vi "Wash Display.vi"(11 "Message Queues":T1) -> ()   [LabVIEW 2017]
uses:
  support/Message Queue/All Message Queues.ctl
  support/Message Queue/Message Cluster.ctl
  Control 1.ctl
  Position Slider.ctl
  support/Message Queue/Message Queue.lvlib
panel:
  out "Wash Entry Display":bool
  out "Vehicle Postion":bool
  out "Air Dry":bool
  out "Tire Shine Foam":bool
  out "Spot Free Rinse":bool
  out "Low Pressure  Wax":bool
  out "High Pressure Wash":bool
  out "Pre-soak":bool
  out "Bug Remover":bool
  out "Under Body Wash":bool
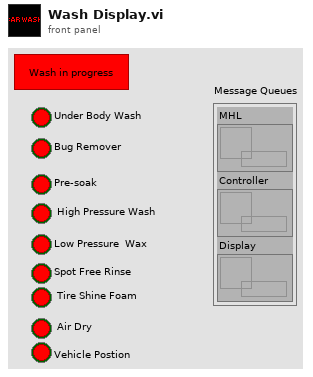
[diagram p1: front panel]
types:
  T1 = typedef "Message Queue.lvlib/All Message Queues.ctl" = cluster{"MHL":refnum<queue>, "Controller":refnum<queue>, "Display":refnum<queue>}
  T2 = typedef "Control 1.ctl" = cluster{"Under Body Wash":bool, "Bug Remover":bool, "Pre-soak":bool, " High Pressure Wash":bool, "Low Pressure  Wax":bool, "Spot Free Rinse":bool, " Tire Shine Foam":bool, " Air Dry":bool, "Vehicle Postion":bool, "Wash Entry Display":bool, "Car Position Slider":T3}
  T3 = typedef "Position Slider.ctl" = i32
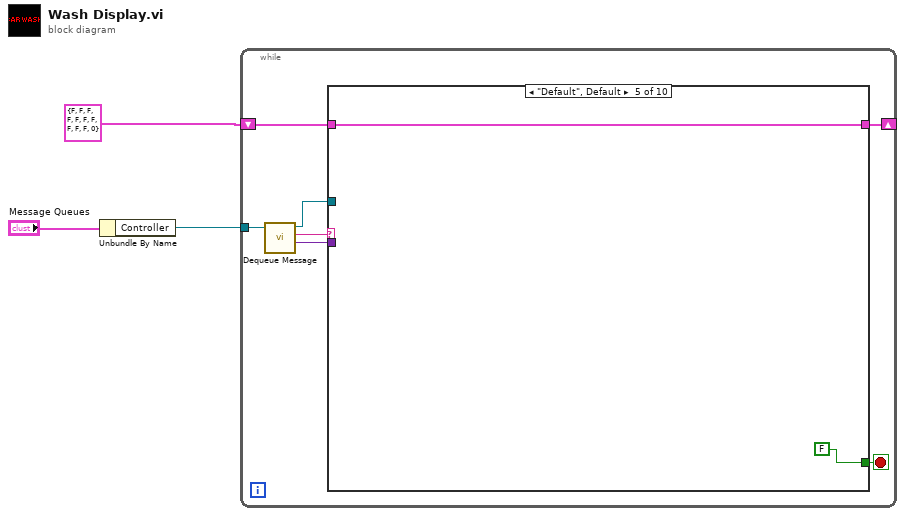
[diagram p0: block diagram]
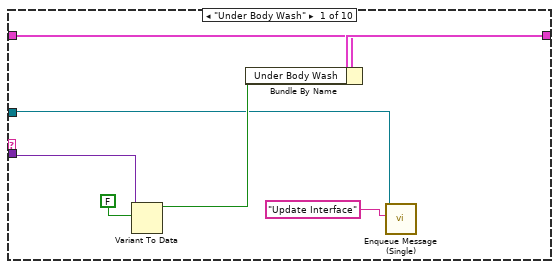
[diagram p2: hidden frame]
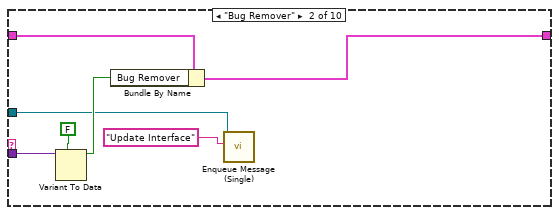
[diagram p3: hidden frame]
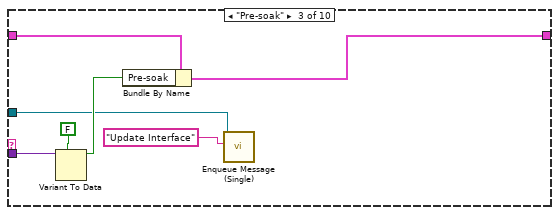
[diagram p4: hidden frame]
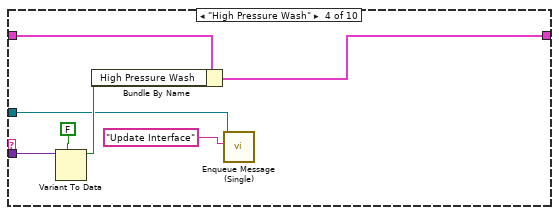
[diagram p5: hidden frame]
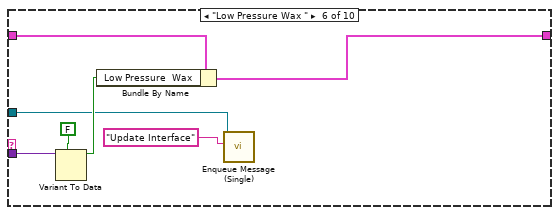
[diagram p6: hidden frame]
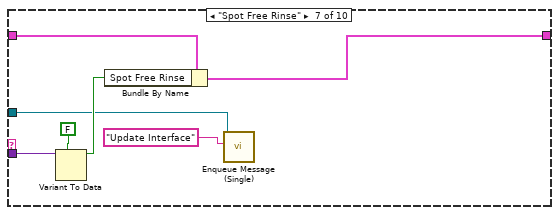
[diagram p7: hidden frame]
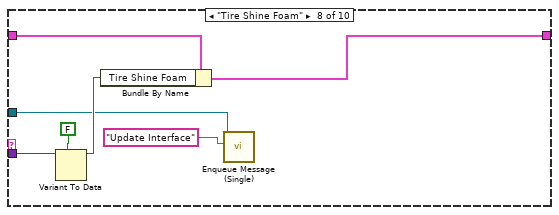
[diagram p8: hidden frame]
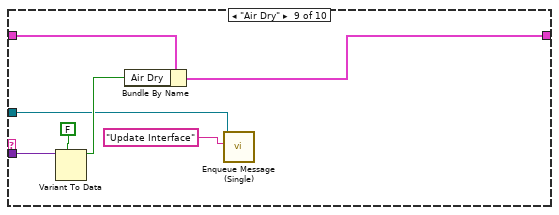
[diagram p9: hidden frame]
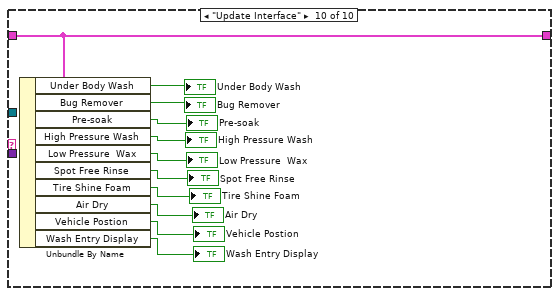
[diagram p10: hidden frame]
diagram:
  n1 = Unbundle By Name("Message Queues") -> ("Controller"=w2:refnum<queue>)
  n2 = while {
    tunnel: w2 -> [w10]
    shift-right: [w7] -> _
    shift-left: T2 {"Under Body Wash"=FALSE, "Bug Remover"=FALSE, "Pre-soak"=FALSE, " High Pressure Wash"=FALSE, "Low Pressure  Wax"=FALSE, "Spot Free Rinse"=FALSE, " Tire Shine Foam"=FALSE, " Air Dry"=FALSE, "Vehicle Postion"=FALSE, "Wash Entry Display"=FALSE, "Car Position Slider"=0} -> [w8]
    stop <- w4 stop-if-true
    n3 = call "Dequeue Message.vi"("Message Queue"=w10) -> ("Message Data"=w5:variant, "Message"=w9:string, "dup Message Queue"=w6:refnum<queue>)  [unwired: 7 in, 1 out]
    n4 = case shown="\"Default\", Default" w9 {
      tunnel: w8 -> [w11 w23 w30 w37 w40 w46 w53 w60 w67 w79]
      tunnel: [w14 w20 w27 w34 w40 w43 w50 w57 w64 w79] -> w7
      tunnel: w6 -> [w13 w19 w26 w33 _ w42 w49 w56 w63 _]
      tunnel: w5 -> [w17 w24 w31 w38 _ w47 w54 w61 w68 _]
      tunnel: [_ _ _ _ FALSE _ _ _ _ _] -> w4
      frame "Under Body Wash" {
        n5 = Variant To Data(type=FALSE, Variant=w17) -> (data=w16:bool)  [unwired: 1 in, 1 out]
        n6 = Bundle By Name(cluster=w11, "Under Body Wash"=w16) -> (w14:T2)
        n7 = call "Enqueue Message (Single).vi"("Message"="Update Interface", "Message Queue"=w13) -> ()  [unwired: 8 in, 2 out]
      }
      frame "Bug Remover" {
        n8 = Variant To Data(type=FALSE, Variant=w24) -> (data=w22:bool)  [unwired: 1 in, 1 out]
        n9 = Bundle By Name(cluster=w23, "Bug Remover"=w22) -> (w20:T2)
        n10 = call "Enqueue Message (Single).vi"("Message"="Update Interface", "Message Queue"=w19) -> ()  [unwired: 8 in, 2 out]
      }
      frame "Pre-soak" {
        n11 = Variant To Data(type=FALSE, Variant=w31) -> (data=w29:bool)  [unwired: 1 in, 1 out]
        n12 = Bundle By Name(cluster=w30, "Pre-soak"=w29) -> (w27:T2)
        n13 = call "Enqueue Message (Single).vi"("Message"="Update Interface", "Message Queue"=w26) -> ()  [unwired: 8 in, 2 out]
      }
      frame "High Pressure Wash" {
        n14 = Variant To Data(type=FALSE, Variant=w38) -> (data=w36:bool)  [unwired: 1 in, 1 out]
        n15 = Bundle By Name(cluster=w37, "High Pressure Wash"=w36) -> (w34:T2)
        n16 = call "Enqueue Message (Single).vi"("Message"="Update Interface", "Message Queue"=w33) -> ()  [unwired: 8 in, 2 out]
      }
      frame "Default", Default {
      }
      frame "Low Pressure Wax " {
        n17 = Variant To Data(type=FALSE, Variant=w47) -> (data=w45:bool)  [unwired: 1 in, 1 out]
        n18 = Bundle By Name(cluster=w46, "Low Pressure  Wax"=w45) -> (w43:T2)
        n19 = call "Enqueue Message (Single).vi"("Message"="Update Interface", "Message Queue"=w42) -> ()  [unwired: 8 in, 2 out]
      }
      frame "Spot Free Rinse" {
        n20 = Variant To Data(type=FALSE, Variant=w54) -> (data=w52:bool)  [unwired: 1 in, 1 out]
        n21 = Bundle By Name(cluster=w53, "Spot Free Rinse"=w52) -> (w50:T2)
        n22 = call "Enqueue Message (Single).vi"("Message"="Update Interface", "Message Queue"=w49) -> ()  [unwired: 8 in, 2 out]
      }
      frame "Tire Shine Foam" {
        n23 = Variant To Data(type=FALSE, Variant=w61) -> (data=w59:bool)  [unwired: 1 in, 1 out]
        n24 = Bundle By Name(cluster=w60, "Tire Shine Foam"=w59) -> (w57:T2)
        n25 = call "Enqueue Message (Single).vi"("Message"="Update Interface", "Message Queue"=w56) -> ()  [unwired: 8 in, 2 out]
      }
      frame "Air Dry" {
        n26 = Variant To Data(type=FALSE, Variant=w68) -> (data=w66:bool)  [unwired: 1 in, 1 out]
        n27 = Bundle By Name(cluster=w67, "Air Dry"=w66) -> (w64:T2)
        n28 = call "Enqueue Message (Single).vi"("Message"="Update Interface", "Message Queue"=w63) -> ()  [unwired: 8 in, 2 out]
      }
      frame "Update Interface" {
        n29 = Unbundle By Name(w79) -> ("Under Body Wash"=→"Under Body Wash":bool, "Bug Remover"=→"Bug Remover":bool, "Pre-soak"=→"Pre-soak":bool, "High Pressure Wash"=→"High Pressure Wash":bool, "Low Pressure  Wax"=→"Low Pressure  Wax":bool, "Spot Free Rinse"=→"Spot Free Rinse":bool, "Tire Shine Foam"=→"Tire Shine Foam":bool, "Air Dry"=→"Air Dry":bool, "Vehicle Postion"=→"Vehicle Postion":bool, "Wash Entry Display"=→"Wash Entry Display":bool)
      }
    }
  }
